vi "Online_Program.vi"() -> ()   [LabVIEW 2014]
uses:
  <vilib>/Utility/file.llb/Read From Spreadsheet File (DBL).vi
  <vilib>/Analysis/Matrix/Numeric/Conversions/Array To Matrix - RA2.vi
  <vilib>/Analysis/Matrix/Numeric/Conversions/Array To Matrix - RA.vi
  <vilib>/Utility/file.llb/Write To Spreadsheet File (DBL).vi
  <vilib>/Utility/file.llb/Write To Spreadsheet File (I64).vi
  <vilib>/Analysis/Matrix/NI_Matrix.lvlib
  <vilib>/Instr/_visa.llb/VISA Configure Serial Port (Instr).vi
  NeuroSky_Dll_Call/Debug/NeuroSky_Dll_Call.dll
panel:
  out "에러 출력":errorcluster
  out "메시지 2":string
  out "큐사인":bool
  out "icon_온도":bool
  out "icon_용변":bool
  out "icon_자판":bool
  out "icon_응급":bool=TRUE
  out "icon_기계":bool
  out "icon_침대":bool
  out "메시지":string
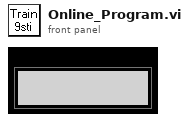
[diagram p1: front panel]
types:
  T1 = typedef "NI_Matrix.lvlib/RealMatrix.ctl" = dbl[][]
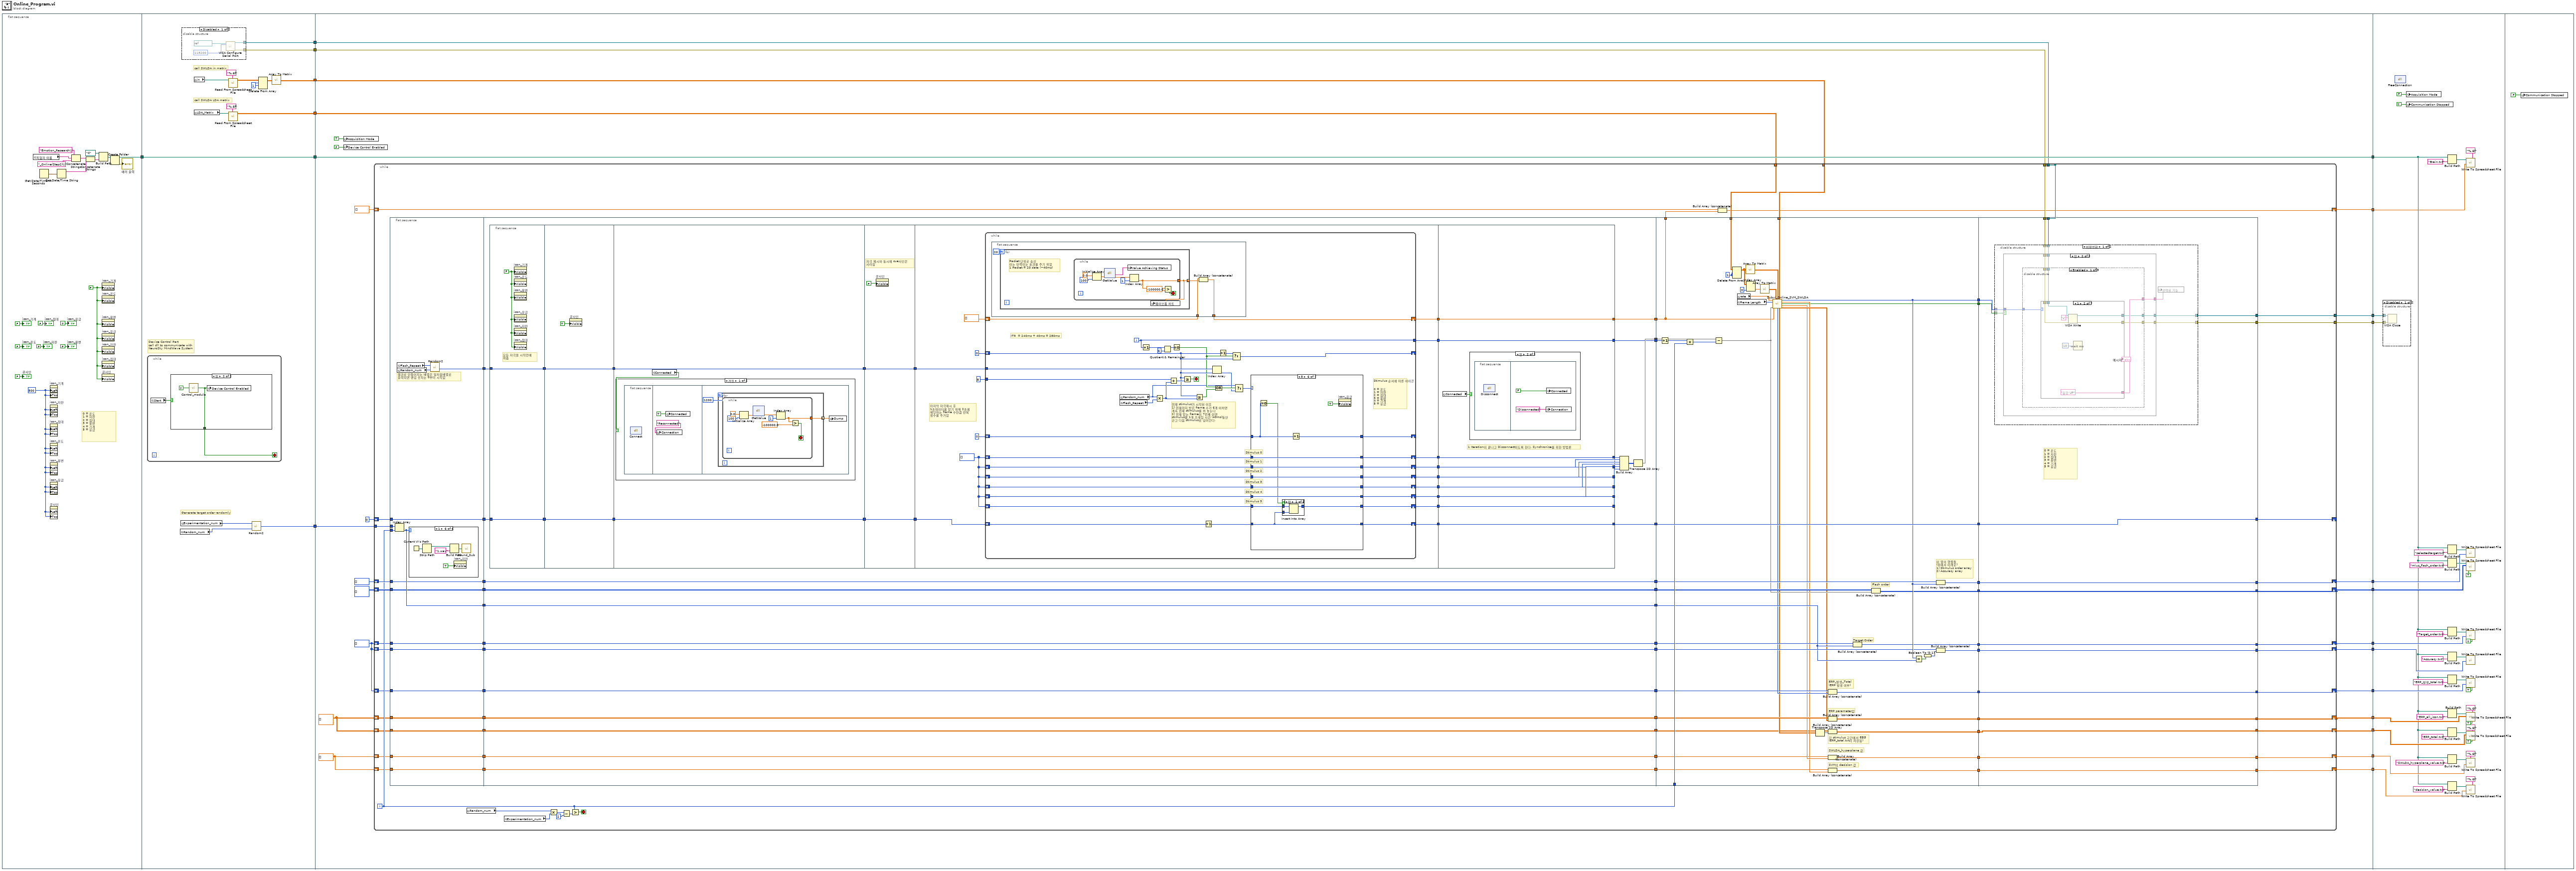
[diagram p0: block diagram]
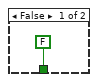
[diagram p3: hidden frame]
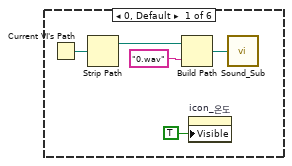
[diagram p4: hidden frame]
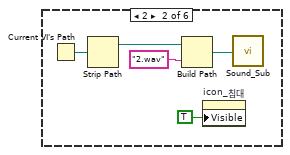
[diagram p5: hidden frame]
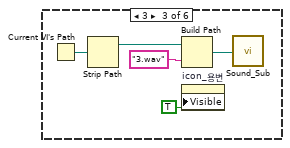
[diagram p6: hidden frame]
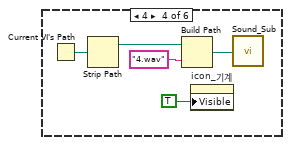
[diagram p7: hidden frame]
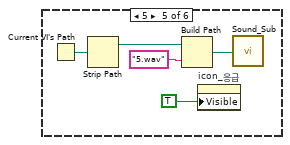
[diagram p8: hidden frame]
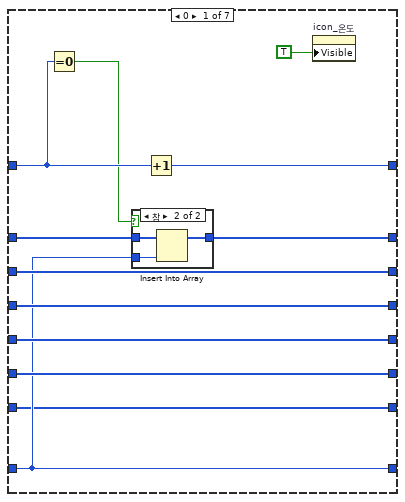
[diagram p10: hidden frame]
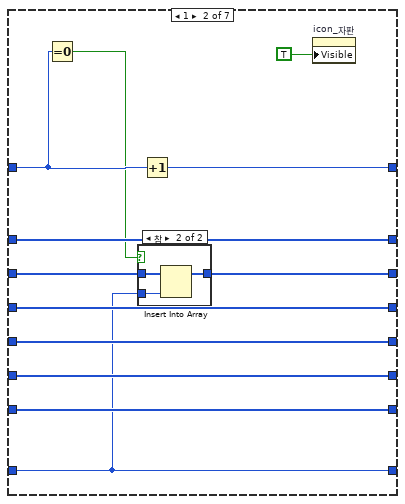
[diagram p12: hidden frame]
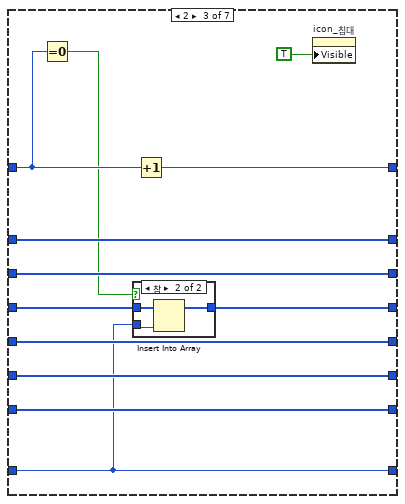
[diagram p14: hidden frame]
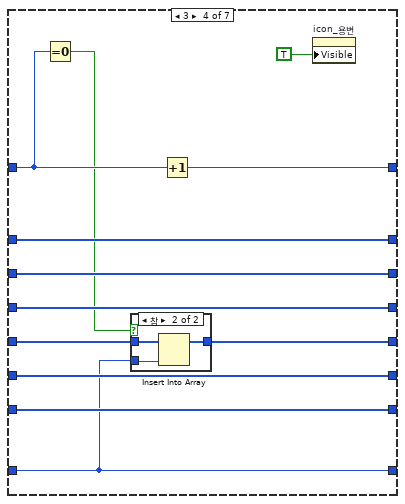
[diagram p16: hidden frame]
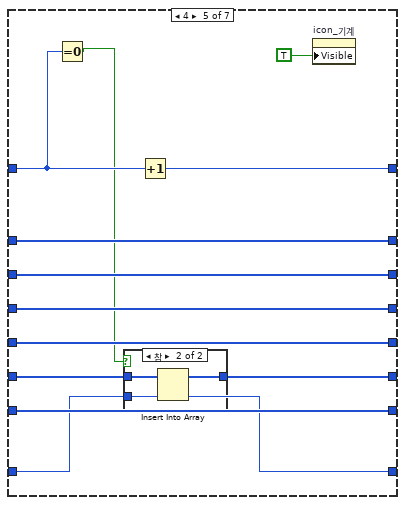
[diagram p18: hidden frame]
diagram:
  n1 = flat-sequence {
    tunnel: [w40] -> w20
    tunnel: w20 -> [w55]
    tunnel: [w55] -> w19
    tunnel: [w53] -> w18
    tunnel: [w49] -> w13
    tunnel: [w43] -> w7
    tunnel: [w42] -> w4
    tunnel: [w41] -> w3
    tunnel: w19 -> [w81]
    tunnel: [w81] -> w17
    tunnel: [w91] -> w16
    tunnel: [w89] -> w15
    tunnel: [w87] -> w14
    tunnel: w18 -> [w70]
    tunnel: w13 -> [w86]
    tunnel: [w85] -> w12
    tunnel: [w82] -> w11
    tunnel: [w78] -> w10
    tunnel: [w76] -> w9
    tunnel: [w75] -> w8
    tunnel: w7 -> [w69]
    tunnel: [w73] -> w6
    tunnel: [w71] -> w5
    tunnel: w4 -> [w68]
    tunnel: w3 -> [w67]
    tunnel: [w66] -> w2
    tunnel: [w65] -> w1
    tunnel: w17 -> [w663]
    tunnel: w16 -> [w658]
    tunnel: w15 -> [w697]
    tunnel: w14 -> [w693]
    tunnel: w12 -> [w690]
    tunnel: w11 -> [w686]
    tunnel: w10 -> [w680]
    tunnel: w9 -> [w675]
    tunnel: w8 -> [w672]
    tunnel: w6 -> [w669]
    tunnel: w5 -> [w664]
    tunnel: w2 -> [w660]
    tunnel: w1 -> [w659]
    frame #0 {
      w22 = FALSE ("Visible")
      w23 = 500 ("Position:Left")
      # "0 = 온도\n1 = 자판\n2 = 침대\n3 = 용변 \n4 = 기계 \n5 = 응급"
      n2 = global read "Control_Panel_정리.vi" "피험자 이름"() -> (w31:string)
      n3 = Get Date/Time In Seconds() -> (seconds since 1Jan1904=w37:timestamp)
      n4 = property on="icon_기계" class="Bool (엄격한)"("Left"=w23, "Top"=w23) -> ()  [unwired: 2 in, 2 out]
      n5 = property on="icon_자판" class="Bool (엄격한)"("Left"=w23, "Top"=w23) -> ()  [unwired: 2 in, 2 out]
      n6 = property on="icon_침대" class="Bool (엄격한)"("Left"=w23, "Top"=w23) -> ()  [unwired: 2 in, 2 out]
      n7 = property on="icon_온도" class="Bool (엄격한)"("Left"=w23, "Top"=w23) -> ()  [unwired: 2 in, 2 out]
      n8 = property on="icon_용변" class="Bool (엄격한)"("Left"=w23, "Top"=w23) -> ()  [unwired: 2 in, 2 out]
      n9 = property on="icon_응급" class="Bool (엄격한)"("Left"=w23, "Top"=w23) -> ()  [unwired: 2 in, 2 out]
      n10 = property on="큐사인" class="Bool (엄격한)"("Left"=w23, "Top"=w23) -> ()  [unwired: 2 in, 2 out]
      n11 = Get Date/Time String(seconds (now)=w37) -> (date string=w38:string)  [unwired: 2 in, 1 out]
      n12 = Concatenate Strings("Emotion_Research\\" ("string"), w31, "_Online(Step2)\\" ("문자열")) -> (w33:string)
      n13 = Concatenate Strings(w33, w38) -> (w35:string)
      n14 = Build Path(base path=path "C:/" ("path"), name or relative path=w35) -> (appended path=w36:path)
      n15 = property on="icon_기계" class="Bool (엄격한)"("Visible"=w22) -> ()  [unwired: 2 in, 2 out]
      n16 = property on="icon_온도" class="Bool (엄격한)"("Visible"=w22) -> ()  [unwired: 2 in, 2 out]
      n17 = property on="icon_용변" class="Bool (엄격한)"("Visible"=w22) -> ()  [unwired: 2 in, 2 out]
      n18 = property on="icon_응급" class="Bool (엄격한)"("Visible"=w22) -> ()  [unwired: 2 in, 2 out]
      n19 = property on="icon_자판" class="Bool (엄격한)"("Visible"=w22) -> ()  [unwired: 2 in, 2 out]
      n20 = property on="icon_침대" class="Bool (엄격한)"("Visible"=w22) -> ()  [unwired: 2 in, 2 out]
      n21 = property on="큐사인" class="Bool (엄격한)"("Visible"=w22) -> ()  [unwired: 2 in, 2 out]
      n22 = Create Folder(path (use dialog)=w36) -> (created path=w40:path, error out=→"에러 출력":errorcluster)  [unwired: 2 in, 1 out]
      "icon_온도" <- FALSE ("icon_전원 6")
      "icon_용변" <- FALSE ("icon_전체종료")
      "icon_자판" <- FALSE ("icon_음량업 2")
      "icon_응급" <- TRUE ("icon_채널다운")
      "icon_기계" <- FALSE ("icon_음량다")
      "icon_침대" <- FALSE ("icon_채널업")
      "큐사인" <- FALSE ("icon_전원 7")
    }
    frame #1 {
      w46 = 1 ("인덱스 (행)")
      # "call SWLDA in matrix"
      # "call SWLDA LDA matrix"
      # "Generate target order randomly"
      # "Device Control Part\ncall dll to communicate with\nNeuroSky MindWave System"
      n23 = while {
        stop <- w61 stop-if-true
        n24 = global read "Control_Panel_정리.vi" "Start"() -> (w60:bool)
        n25 = case shown="참" w60 {
          tunnel: [FALSE ("Connected") w63] -> w61
          frame False {
          }
          frame True {
            n26 = call "Control_module.vi"("Turn on"=TRUE ("Device Control Enabled")) -> ("Connected"=w63:bool)
            n27 = global write "Control_Panel_정리.vi" "Device Control Enabled"(w63) -> ()
          }
        }
      }
      n28 = global read "Control_Panel_정리.vi" "Random_num"() -> (w50:i32)
      n29 = global read "Control_Panel_정리.vi" "Experimentation_num"() -> (w51:i32)
      n30 = disable-structure shown="Disabled" {
        disable-tunnel: [w57 _] -> w42
        disable-tunnel: [w56 _] -> w41
        frame Disabled {
          n31 = call-poly "VISA Configure Serial Port"("VISA resource name"=refnum<visa-resource-name> "COM3", "baud rate (9600)"=u32 115200) -> ("VISA resource name out"=w57:refnum<visa-resource-name>, "error out"=w56:errorcluster)  [unwired: 12 in]
        }
        frame Enabled {
        }
      }
      n32 = global read "Control_Panel_정리.vi" "in"() -> (w44:path)
      n33 = global read "Control_Panel_정리.vi" "LDA_Matrix"() -> (w52:path)
      n34 = call-poly <vilib>:"Read From Spreadsheet File.vi"("format (%.3f)"="%.6f", "file path (dialog if empty)"=w44) -> ("all rows"=w45:dbl[][])  [unwired: 5 in, 4 out]
      n35 = call-poly <vilib>:"Read From Spreadsheet File.vi"("format (%.3f)"="%.6f", "file path (dialog if empty)"=w52) -> ("all rows"=w53:dbl[][])  [unwired: 5 in, 4 out]
      n36 = call "Random2.vi"("Random_num"=w50, "전체횟수"=w51) -> ("배열"=w49:i32[])
      n37 = Delete From Array(array=w45, length=w46, index (row)=w46) -> (array with subset deleted=w47:dbl[][])  [unwired: 1 in, 1 out]
      n38 = call-poly <vilib>:"Array To Matrix.vi"("Real 2D Array"=w47) -> ("Real Matrix"=w43:T1)
    }
    frame #2 {
      w74 = dbl[] []
      w72 = dbl[][] []
      w77 = i16[] []
      n39 = global write "Control_Panel_정리.vi" "Acquisition Mode"(TRUE ("Device Control Enabled")) -> ()
      n40 = global write "Control_Panel_정리.vi" "Device Control Enabled"(FALSE ("Device Control Enabled")) -> ()
      n41 = while {
        shift-right: [w92] -> w91
        shift-left: dbl[] [] -> [w100]
        shift-right: [w159] -> _
        shift-left: 0 ("y") -> [w165]
        shift-right: [w134] -> w89
        shift-left: i32[][] [] -> [w137]
        shift-right: [w143] -> w87
        shift-left: i32[] [] -> [w147]
        tunnel: w86 -> [w156]
        shift-right: [w138] -> w85
        shift-left: w77 -> [w142]
        shift-right: [w127] -> w82
        shift-left: w77 -> [w129]
        shift-right: [w125] -> w78
        shift-left: w77 -> [w124]
        shift-right: [w120] -> w76
        shift-left: w72 -> [w119]
        shift-right: [w115] -> w75
        shift-left: w74 -> [w114]
        shift-right: [w110] -> w73
        shift-left: w74 -> [w109]
        shift-right: [w105] -> w71
        shift-left: w72 -> [w104]
        tunnel: w70 -> [w101]
        tunnel: w69 -> [w98]
        tunnel: [w95] -> _
        tunnel: w68 -> [w95]
        tunnel: w67 -> [w96]
        tunnel: [w94] -> w66
        tunnel: [w93] -> w65
        i -> [w132]
        stop <- w148 stop-if-true
        n42 = flat-sequence {
          tunnel: [w182] -> w166
          tunnel: w165 -> [w181]
          tunnel: [w181] -> w164
          tunnel: w156 -> [w180]
          tunnel: w132 -> [w179]
          tunnel: [w176] -> w155
          tunnel: w147 -> [w175]
          tunnel: [w175] -> w146
          tunnel: w142 -> [w174]
          tunnel: [w174] -> w140
          tunnel: w137 -> [w173]
          tunnel: [w173] -> w135
          tunnel: [w172] -> w130
          tunnel: w129 -> [w172]
          tunnel: w124 -> [w171]
          tunnel: [w171] -> w122
          tunnel: w119 -> [w170]
          tunnel: [w170] -> w117
          tunnel: w114 -> [w169]
          tunnel: [w169] -> w112
          tunnel: w109 -> [w168]
          tunnel: [w168] -> w107
          tunnel: w104 -> [w167]
          tunnel: [w167] -> w103
          tunnel: w166 -> [w252]
          tunnel: w164 -> [w249]
          tunnel: [w250] -> w163
          tunnel: [w239] -> w162
          tunnel: [w248] -> w161
          tunnel: [w247] -> w160
          tunnel: w155 -> [w246]
          tunnel: [w246] -> w154
          tunnel: w146 -> [w245]
          tunnel: [w245] -> w145
          tunnel: [w244] -> w141
          tunnel: w140 -> [w244]
          tunnel: [w243] -> w136
          tunnel: w135 -> [w243]
          tunnel: [w242] -> w131
          tunnel: w130 -> [w242]
          tunnel: [w241] -> w123
          tunnel: w122 -> [w241]
          tunnel: [w240] -> w118
          tunnel: w117 -> [w240]
          tunnel: [w238] -> w113
          tunnel: w112 -> [w238]
          tunnel: [w237] -> w108
          tunnel: w107 -> [w237]
          tunnel: w103 -> [w236]
          tunnel: [w236] -> w102
          tunnel: w163 -> [w491]
          tunnel: w162 -> [w465]
          tunnel: w161 -> [w505]
          tunnel: w160 -> [w506]
          tunnel: w132 -> [w504]
          tunnel: [w505] -> w158
          tunnel: [w499] -> w157
          tunnel: w154 -> [w490]
          tunnel: w145 -> [w500]
          tunnel: [w498] -> w144
          tunnel: w141 -> [w496]
          tunnel: [w495] -> w139
          tunnel: w136 -> [w494]
          tunnel: [w492] -> w133
          tunnel: w131 -> [w489]
          tunnel: [w488] -> w128
          tunnel: [w486] -> w126
          tunnel: w123 -> [w485]
          tunnel: [w483] -> w121
          tunnel: w118 -> [w482]
          tunnel: [w480] -> w116
          tunnel: w113 -> [w479]
          tunnel: [w477] -> w111
          tunnel: w108 -> [w476]
          tunnel: [w473] -> w106
          tunnel: w102 -> [w472]
          tunnel: w101 -> [w471]
          tunnel: [w465] -> w99
          tunnel: w98 -> [w467]
          tunnel: [w466] -> w97
          tunnel: [w527] -> w159
          tunnel: [w526] -> w143
          tunnel: [w523] -> w138
          tunnel: [w525] -> w134
          tunnel: [w524] -> w127
          tunnel: [w522] -> w125
          tunnel: [w521] -> w120
          tunnel: [w520] -> w115
          tunnel: [w519] -> w110
          tunnel: [w518] -> w105
          tunnel: w106 -> [w518]
          tunnel: w111 -> [w519]
          tunnel: w116 -> [w520]
          tunnel: w121 -> [w521]
          tunnel: w126 -> [w522]
          tunnel: w128 -> [w524]
          tunnel: w133 -> [w525]
          tunnel: w139 -> [w523]
          tunnel: w144 -> [w526]
          tunnel: w157 -> [w517]
          tunnel: w158 -> [w527]
          tunnel: w97 -> [w516]
          tunnel: w96 -> [w515]
          tunnel: w95 -> [w514]
          tunnel: [w513] -> w94
          tunnel: [w512] -> w93
          frame #0 {
            # "결과로 만들어지는 배열은 일차원배열로\n출력되면 랜덤 숫자는 0부터 시작함"
            n43 = Index Array(array=w180, index=w179) -> (element=w176:i32)
            n44 = global read "Control_Panel_정리.vi" "Flash_Repeat"() -> (w178:i32)
            n45 = global read "Control_Panel_정리.vi" "Random_num"() -> (w177:i32)
            n46 = case shown="1" w176 {
              frame 0, Default {
                n47 = Current VI's Path() -> (path=w185:path)
                n48 = Strip Path(path=w185) -> (stripped path=w186:path)  [unwired: 1 out]
                n49 = Build Path(base path=w186, name or relative path="0.wav" ("이름 또는 상대 경로")) -> (appended path=w184:path)
                n50 = property on="icon_온도" class="Bool (엄격한)"("Visible"=TRUE) -> ()  [unwired: 2 in, 2 out]
                n51 = call "Sound_Sub.vi"("path"=w184) -> ()
              }
              frame 2 {
                n52 = Current VI's Path() -> (path=w189:path)
                n53 = Strip Path(path=w189) -> (stripped path=w190:path)  [unwired: 1 out]
                n54 = Build Path(base path=w190, name or relative path="2.wav" ("이름 또는 상대 경로")) -> (appended path=w192:path)
                n55 = property on="icon_침대" class="Bool (엄격한)"("Visible"=TRUE) -> ()  [unwired: 2 in, 2 out]
                n56 = call "Sound_Sub.vi"("path"=w192) -> ()
              }
              frame 3 {
                n57 = Current VI's Path() -> (path=w194:path)
                n58 = Strip Path(path=w194) -> (stripped path=w195:path)  [unwired: 1 out]
                n59 = Build Path(base path=w195, name or relative path="3.wav" ("이름 또는 상대 경로")) -> (appended path=w197:path)
                n60 = property on="icon_용변" class="Bool (엄격한)"("Visible"=TRUE) -> ()  [unwired: 2 in, 2 out]
                n61 = call "Sound_Sub.vi"("path"=w197) -> ()
              }
              frame 4 {
                n62 = Current VI's Path() -> (path=w199:path)
                n63 = Strip Path(path=w199) -> (stripped path=w200:path)  [unwired: 1 out]
                n64 = Build Path(base path=w200, name or relative path="4.wav" ("이름 또는 상대 경로")) -> (appended path=w202:path)
                n65 = property on="icon_기계" class="Bool (엄격한)"("Visible"=TRUE) -> ()  [unwired: 2 in, 2 out]
                n66 = call "Sound_Sub.vi"("path"=w202) -> ()
              }
              frame 5 {
                n67 = Current VI's Path() -> (path=w204:path)
                n68 = Strip Path(path=w204) -> (stripped path=w205:path)  [unwired: 1 out]
                n69 = Build Path(base path=w205, name or relative path="5.wav" ("이름 또는 상대 경로")) -> (appended path=w207:path)
                n70 = property on="icon_응급" class="Bool (엄격한)"("Visible"=TRUE) -> ()  [unwired: 2 in, 2 out]
                n71 = call "Sound_Sub.vi"("path"=w207) -> ()
              }
              frame 1 {
                n72 = Current VI's Path() -> (path=w210:path)
                n73 = Strip Path(path=w210) -> (stripped path=w211:path)  [unwired: 1 out]
                n74 = Build Path(base path=w211, name or relative path="1.wav" ("이름 또는 상대 경로")) -> (appended path=w209:path)
                n75 = property on="icon_자판" class="Bool (엄격한)"("Visible"=TRUE) -> ()  [unwired: 2 in, 2 out]
                n76 = call "Sound_Sub.vi"("path"=w209) -> ()
              }
            }
            n77 = call "Random2.vi"("Random_num"=w177, "전체횟수"=w178) -> ("배열"=w182:i32[])
          }
          frame #1 {
            n78 = flat-sequence {
              tunnel: w249 -> [w254]
              tunnel: w252 -> [w255]
              tunnel: [w255] -> w235
              tunnel: [w254] -> w234
              tunnel: [w258] -> w227
              tunnel: [w257] -> w226
              tunnel: w235 -> [w258]
              tunnel: w234 -> [w257]
              tunnel: w227 -> [w261]
              tunnel: [w261] -> w216
              tunnel: w226 -> [w260]
              tunnel: [w260] -> w214
              tunnel: w216 -> [w277]
              tunnel: [w277] -> w215
              tunnel: w214 -> [w276]
              tunnel: [w276] -> w213
              tunnel: w215 -> [w293]
              tunnel: w213 -> [w283]
              tunnel: [w291] -> w225
              tunnel: [w290] -> w224
              tunnel: [w289] -> w223
              tunnel: [w288] -> w222
              tunnel: [w287] -> w221
              tunnel: [w282] -> w220
              tunnel: [w281] -> w219
              tunnel: [w280] -> w218
              tunnel: [w278] -> w217
              tunnel: [w454] -> w239
              tunnel: [w455] -> w230
              tunnel: [w456] -> w247
              tunnel: [w457] -> w248
              tunnel: [w458] -> w233
              tunnel: [w459] -> w232
              tunnel: [w460] -> w231
              tunnel: [w461] -> w229
              tunnel: [w462] -> w228
              tunnel: w225 -> [w462]
              tunnel: w224 -> [w461]
              tunnel: w223 -> [w460]
              tunnel: w222 -> [w459]
              tunnel: w221 -> [w458]
              tunnel: w220 -> [w457]
              tunnel: w219 -> [w456]
              tunnel: w218 -> [w455]
              tunnel: w217 -> [w454]
              frame #0 {
                w253 = FALSE ("Visible")
                # "모든 자극을 시작전에\n꺼줌"
                n79 = property on="icon_기계" class="Bool (엄격한)"("Visible"=w253) -> ()  [unwired: 2 in, 2 out]
                n80 = property on="icon_온도" class="Bool (엄격한)"("Visible"=w253) -> ()  [unwired: 2 in, 2 out]
                n81 = property on="icon_용변" class="Bool (엄격한)"("Visible"=w253) -> ()  [unwired: 2 in, 2 out]
                n82 = property on="icon_응급" class="Bool (엄격한)"("Visible"=w253) -> ()  [unwired: 2 in, 2 out]
                n83 = property on="icon_자판" class="Bool (엄격한)"("Visible"=w253) -> ()  [unwired: 2 in, 2 out]
                n84 = property on="icon_침대" class="Bool (엄격한)"("Visible"=w253) -> ()  [unwired: 2 in, 2 out]
              }
              frame #1 {
                n85 = property on="큐사인" class="Bool (엄격한)"("Visible"=TRUE) -> ()  [unwired: 2 in, 2 out]
              }
              frame #2 {
                n86 = global read "Control_Panel_정리.vi" "Connected"() -> (w259:bool)
                n87 = case shown="거짓" w259 {
                  frame False {
                    n88 = flat-sequence {
                      frame #0 {
                        n89 = dll-call lib="C:/Users/Server/Desktop/NeuroSky/NeuroSky_Dll_Call/Debug/NeuroSky_Dll_Call.dll" fn="Connect"() -> ()  [unwired: 4 in, 2 out]
                      }
                      frame #1 {
                        n90 = global write "Control_Panel_정리.vi" "Connection"("Reconnected") -> ()
                        n91 = global write "Control_Panel_정리.vi" "Connected"(TRUE ("Connected")) -> ()
                      }
                      frame #2 {
                        n92 = for {
                          N: 1200 -> [_]
                          tunnel: [w266] -> w264 mode=indexing
                          n93 = while {
                            tunnel: [w268] -> w266
                            stop <- w267 stop-if-true
                            n94 = Initialize Array(0.0 ("element"), 100 ("dimension size")) -> (w273:dbl[])
                            n95 = dll-call lib="C:/Users/Server/Desktop/NeuroSky/NeuroSky_Dll_Call/Debug/NeuroSky_Dll_Call.dll" fn="GetValue"("result"=w273) -> ("result"=w274:dbl[])  [unwired: 4 in, 2 out]
                            n96 = Index Array(array=w274, index=1) -> (element=w268:dbl)
                            n97 = Greater?(x=w268, y=-100000.0) -> (0:w267:bool)
                          }
                        }
                        n98 = global write "Control_Panel_정리.vi" "Dump"(w264) -> ()
                      }
                    }
                  }
                  frame True {
                  }
                }
              }
              frame #3 {
                # "자극 제시와 동시에 cue사인은\n사라짐"
                n99 = property on="큐사인" class="Bool (엄격한)"("Visible"=FALSE) -> ()  [unwired: 2 in, 2 out]
              }
              frame #4 {
                w285 = i32[] []
                # "마지막 자극제시 후\n1초데이터를 받기 위해 2초에\n해당하는 frame 수만큼 반복\n횟수를 추가함"
                n100 = while {
                  tunnel: w293 -> [w329]
                  shift-right: [w297] -> w278
                  shift-left: dbl[] [] -> [w298]
                  tunnel: 8 -> [w294]
                  shift-right: [w326] -> w291
                  shift-left: w285 -> [w325]
                  shift-right: [w323] -> w290
                  shift-left: w285 -> [w324]
                  shift-right: [w321] -> w280
                  shift-left: w285 -> [w322]
                  shift-right: [w319] -> w289
                  shift-left: w285 -> [w320]
                  shift-right: [w317] -> w288
                  shift-left: w285 -> [w318]
                  shift-right: [w316] -> w287
                  shift-left: w285 -> [w303]
                  shift-right: [w314] -> w282
                  shift-left: w283 -> [w315]
                  shift-right: [w310] -> _
                  shift-left: 0 -> [w309]
                  shift-right: [w304] -> _
                  shift-left: 0 ("y") -> [w305]
                  tunnel: [w299] -> w281
                  i -> [w299]
                  stop <- w330 stop-if-true
                  # "ITR  = 240ms + 40ms = 280ms"
                  # "현재 stimulus가 시작된 이후\n1) 현재까지 받은 frame 수가 6개 이하면\n계속 현재 stimulus를 켜 놓는다\n2) 현재 받는 frame이 7번째 이면\nstimulus를 1개 프레임 시간 (40ms)동안\n끈고 다음 stimulus로 넘어간다."
                  # "Stimulus 순서에 따른 아이콘\n\n\n0 = 온도\n1 = 자판\n2 = 침대\n3 = 용변 \n4 = 기계 \n5 = 응급"
                  # "Stimulus 5"
                  # "Stimulus 4"
                  # "Stimulus 3"
                  # "Stimulus 2"
                  # "Stimulus 1"
                  # "Stimulus 0"
                  n101 = flat-sequence {
                    tunnel: [w335] -> w297
                    tunnel: w298 -> [w334]
                    frame #0 {
                      n102 = for {
                        N: 20 -> [_]
                        tunnel: [w336] -> w333 mode=indexing
                        # "Packet 단위로 송신\n이는 반짝이는 효과를 주기 위함\n1 Packet = 20 data (~40ms)"
                        n103 = while {
                          tunnel: [w338] -> w336
                          stop <- w337 stop-if-true
                          n104 = Initialize Array(0.0 ("element"), 100 ("dimension size")) -> (w344:dbl[])
                          n105 = dll-call lib="C:/Users/Server/Desktop/NeuroSky/NeuroSky_Dll_Call/Debug/NeuroSky_Dll_Call.dll" fn="GetValue"("result"=w344) -> ("errCode"=w340:string, "result"=w345:dbl[])  [unwired: 3 in, 2 out]
                          n106 = global write "Control_Panel_정리.vi" "Value Achieving Status"(w340) -> ()
                          n107 = Index Array(array=w345, index=1) -> (element=w338:dbl)
                          n108 = Greater?(x=w338, y=-100000.0) -> (0:w337:bool)
                        }
                        n109 = global write "Control_Panel_정리.vi" "웨이브폼 차트"(w336) -> ()
                      }
                      n110 = Build Array (concatenate)(w334, w333) -> (w335:dbl[])
                    }
                  }
                  n111 = global read "Control_Panel_정리.vi" "Random_num"() -> (w296:i32)
                  n112 = global read "Control_Panel_정리.vi" "Flash_Repeat"() -> (w295:i32)
                  n113 = Increment(x=w299) -> (x+1=w302:i32)
                  n114 = Multiply(x=w296, y=w295) -> (x*y=w300:i32)
                  n115 = Quotient & Remainder(x=w302, y=6) -> (x-y*floor(x/y)=w312:i32)  [unwired: 1 out]
                  n116 = Add(x=w294, y=w300) -> (x+y=w331:i32)
                  n117 = Equal To 0?(x=w312) -> (x = 0?=w308:bool)
                  n118 = Greater Or Equal?(x=w309, y=w331) -> (x >= y?=w330:bool)
                  n119 = Greater Or Equal?(x=w309, y=w300) -> (x >= y?=w307:bool)
                  n120 = Increment(x=w315) -> (x+1=w327:i32)
                  n121 = Index Array(array=w329, index=w309) -> (element=w301:i32)
                  n122 = Or(x=w308, y=w307) -> (x .or. y?=w306:bool)
                  n123 = Increment(x=w309) -> (x+1=w311:i32)
                  n124 = Select(t=w311, s=w308, f=w309) -> (s? t:f=w310:i32)
                  n125 = Select(t=w296, s=w306, f=w301) -> (s? t:f=w328:i32)
                  n126 = case shown="5" w328 {
                    tunnel: w327 -> [w351 w367 w382 w398 w414 w431 w446]
                    tunnel: [w356 w364 w389 w405 w421 w437 w452] -> w326
                    tunnel: w325 -> [w357 w364 w389 w405 w421 w437 w452]
                    tunnel: w324 -> [w355 w373 w386 w402 w418 w435 w451]
                    tunnel: [w355 w372 w386 w402 w418 w435 w451] -> w323
                    tunnel: w322 -> [w354 w371 w388 w401 w417 w434 w450]
                    tunnel: [w354 w371 w387 w401 w417 w434 w450] -> w321
                    tunnel: w320 -> [w353 w370 w385 w404 w416 w433 w449]
                    tunnel: [w353 w370 w385 w403 w416 w433 w449] -> w319
                    tunnel: w318 -> [w352 w369 w384 w400 w420 w432 w448]
                    tunnel: [w352 w369 w384 w400 w419 w432 w448] -> w317
                    tunnel: w303 -> [w348 w368 w383 w399 w415 w436 w447]
                    tunnel: [w348 w368 w383 w399 w415 w428 w447] -> w316
                    tunnel: [w351 w367 w382 w398 w414 w431 w446] -> w314
                    tunnel: w305 -> [w350 w366 w381 w396 w413 w429 _]
                    tunnel: [w349 w365 w380 w397 w412 w430 0] -> w304
                    frame 0 {
                      n127 = Equal To 0?(x=w350) -> (x = 0?=w346:bool)
                      n128 = case shown="참" w346 {
                        tunnel: w357 -> [w358 w361]
                        tunnel: [w358 w360] -> w356
                        tunnel: w351 -> [_ w359]
                        frame False {
                        }
                        frame True {
                          n129 = Insert Into Array(array=w361, new element=w359) -> (w360:i32[])  [unwired: 1 in]
                        }
                      }
                      n130 = Increment(x=w350) -> (x+1=w349:i32)
                      n131 = property on="icon_온도" class="Bool (엄격한)"("Visible"=TRUE) -> ()  [unwired: 2 in, 2 out]
                    }
                    frame 1 {
                      n132 = Equal To 0?(x=w366) -> (x = 0?=w362:bool)
                      n133 = case shown="참" w362 {
                        tunnel: w373 -> [w374 w377]
                        tunnel: [w374 w376] -> w372
                        tunnel: w367 -> [_ w375]
                        frame False {
                        }
                        frame True {
                          n134 = Insert Into Array(array=w377, new element=w375) -> (w376:i32[])  [unwired: 1 in]
                        }
                      }
                      n135 = Increment(x=w366) -> (x+1=w365:i32)
                      n136 = property on="icon_자판" class="Bool (엄격한)"("Visible"=TRUE) -> ()  [unwired: 2 in, 2 out]
                    }
                    frame 2 {
                      n137 = Equal To 0?(x=w381) -> (x = 0?=w378:bool)
                      n138 = case shown="참" w378 {
                        tunnel: w388 -> [w390 w393]
                        tunnel: [w390 w392] -> w387
                        tunnel: w382 -> [_ w391]
                        frame False {
                        }
                        frame True {
                          n139 = Insert Into Array(array=w393, new element=w391) -> (w392:i32[])  [unwired: 1 in]
                        }
                      }
                      n140 = Increment(x=w381) -> (x+1=w380:i32)
                      n141 = property on="icon_침대" class="Bool (엄격한)"("Visible"=TRUE) -> ()  [unwired: 2 in, 2 out]
                    }
                    frame 3 {
                      n142 = Equal To 0?(x=w396) -> (x = 0?=w394:bool)
                      n143 = case shown="참" w394 {
                        tunnel: w404 -> [w406 w409]
                        tunnel: [w406 w408] -> w403
                        tunnel: w398 -> [_ w407]
                        frame False {
                        }
                        frame True {
                          n144 = Insert Into Array(array=w409, new element=w407) -> (w408:i32[])  [unwired: 1 in]
                        }
                      }
                      n145 = Increment(x=w396) -> (x+1=w397:i32)
                      n146 = property on="icon_용변" class="Bool (엄격한)"("Visible"=TRUE) -> ()  [unwired: 2 in, 2 out]
                    }
                    frame 4 {
                      n147 = Equal To 0?(x=w413) -> (x = 0?=w410:bool)
                      n148 = case shown="참" w410 {
                        tunnel: w420 -> [w422 w425]
                        tunnel: [w422 w424] -> w419
                        tunnel: w414 -> [_ w423]
                        frame False {
                        }
                        frame True {
                          n149 = Insert Into Array(array=w425, new element=w423) -> (w424:i32[])  [unwired: 1 in]
                        }
                      }
                      n150 = Increment(x=w413) -> (x+1=w412:i32)
                      n151 = property on="icon_기계" class="Bool (엄격한)"("Visible"=TRUE) -> ()  [unwired: 2 in, 2 out]
                    }
                    frame 5 {
                      n152 = Equal To 0?(x=w429) -> (x = 0?=w426:bool)
                      n153 = case shown="참" w426 {
                        tunnel: w436 -> [w438 w441]
                        tunnel: [w438 w440] -> w428
                        tunnel: w431 -> [_ w439]
                        frame False {
                        }
                        frame True {
                          n154 = Insert Into Array(array=w441, new element=w439) -> (w440:i32[])  [unwired: 1 in]
                        }
                      }
                      n155 = Increment(x=w429) -> (x+1=w430:i32)
                      n156 = property on="icon_응급" class="Bool (엄격한)"("Visible"=TRUE) -> ()  [unwired: 2 in, 2 out]
                    }
                    frame 6, Default {
                      w443 = FALSE ("Visible")
                      w444 = FALSE ("Visible")
                      w442 = FALSE ("Visible")
                      n157 = property on="icon_기계" class="Bool (엄격한)"("Visible"=w442) -> ()  [unwired: 2 in, 2 out]
                      n158 = property on="icon_온도" class="Bool (엄격한)"("Visible"=w442) -> ()  [unwired: 2 in, 2 out]
                      n159 = property on="icon_응급" class="Bool (엄격한)"("Visible"=w444) -> ()  [unwired: 2 in, 2 out]
                      n160 = property on="icon_용변" class="Bool (엄격한)"("Visible"=w444) -> ()  [unwired: 2 in, 2 out]
                      n161 = property on="icon_자판" class="Bool (엄격한)"("Visible"=w443) -> ()  [unwired: 2 in, 2 out]
                      n162 = property on="icon_침대" class="Bool (엄격한)"("Visible"=w443) -> ()  [unwired: 2 in, 2 out]
                    }
                  }
                }
              }
              frame #5 {
                # "1 Iteration이 끝나고 Disconnect하도록 한다. Synchronize를 위한 방법론"
                n163 = global read "Control_Panel_정리.vi" "Connected"() -> (w453:bool)
                n164 = case shown="참" w453 {
                  frame False {
                  }
                  frame True {
                    n165 = flat-sequence {
                      frame #0 {
                        n166 = dll-call lib="C:/Users/Server/Desktop/NeuroSky/NeuroSky_Dll_Call/Debug/NeuroSky_Dll_Call.dll" fn="Disconnect"() -> ()  [unwired: 4 in, 2 out]
                      }
                      frame #1 {
                        n167 = global write "Control_Panel_정리.vi" "Connection"("Disconnected") -> ()
                        n168 = global write "Control_Panel_정리.vi" "Connected"(FALSE ("Connected")) -> ()
                      }
                    }
                  }
                }
              }
            }
            n169 = Build Array(w228, w229, w230, w231, w232, w233) -> (w251:i32[][])
            n170 = Transpose 2D Array(2D array=w251) -> (transposed array=w250:i32[][])
          }
          frame #2 {
            w509 = 1 ("인덱스 (행)")
            # "각 stimulus 구간에서 EEG\n(ERP_total.txt라 저장됨)"
            # "ERP parameter값"
            # "SVM의 decision 값"
            # "SWLDA_hyperplane 값"
            # "ERP_발생_Total\n(ERP 발생 여부)"
            # "Target Order"
            # "Flash order"
            # "이 열의 행렬들 \n(위에서 아래로)\n1) Stimulus order array\n2) Accuracy array"
            n171 = Increment(x=w506) -> (x+1=w510:i32)
            n172 = Multiply(x=w510, y=w504) -> (x*y=w511:i32)
            n173 = Subtract(x=w491, y=w511) -> (x-y=w493:i32[][])
            n174 = Delete From Array(array=w471, length=w509, index (row)=w509) -> (array with subset deleted=w469:dbl[][])  [unwired: 1 in, 1 out]
            n175 = global read "Control_Panel_정리.vi" "rate"() -> (w502:dbl)
            n176 = global read "Control_Panel_정리.vi" "Frame Length"() -> (w503:i32)
            n177 = call-poly <vilib>:"Array To Matrix.vi"("Real 2D Array"=w469) -> ("Real Matrix"=w468:T1)
            n178 = Index Array(array=w469, index (col)=0 ("인덱스")) -> (element=w470:dbl[])  [unwired: 1 in]
            n179 = call-poly <vilib>:"Array To Matrix.vi"("Real 1D Array"=w470) -> ("Real Matrix (Column Vector)"=w507:T1)
            n180 = call "Subvi_Online_SVM_SWLDA.vi"("rate"=w502, "Value"=w507, "Matrix"=w468, "in"=w467, "samples per channel"=w503, "Brain_data_source"=w465, "Target_Flash_Order"=w493) -> ("output-0~8"=w499:i32, "decision"=w478:dbl[], "ERP_발생여부"=w466:bool, "SWLDA"=w481:dbl[], "EPR_발생_total"=w487:i16[], "ERP_all"=w475:dbl[][], "ERP_Parameters"=w484:dbl[][])  [unwired: 2 in]
            n181 = Transpose 2D Array(2D array=w475) -> (transposed array=w474:dbl[][])
            n182 = Build Array (concatenate)(w485, w487) -> (w486:i16[])
            n183 = Build Array (concatenate)(w482, w484) -> (w483:dbl[][])
            n184 = Build Array (concatenate)(w472, w474) -> (w473:dbl[][])
            n185 = Build Array (concatenate)(w479, w481) -> (w480:dbl[])
            n186 = Build Array (concatenate)(w476, w478) -> (w477:dbl[])
            n187 = Build Array (concatenate)(w489, w490) -> (w488:i32[])
            n188 = Build Array (concatenate)(w494, w493) -> (w492:i32[][])
            n189 = Equal?(x=w499, y=w490) -> (x = y?=w501:bool)
            n190 = Boolean To (0,1)(Boolean=w501) -> (0, 1=w497:i16)
            n191 = Build Array (concatenate)(w500, w499) -> (w498:i32[])
            n192 = Build Array (concatenate)(w496, w497) -> (w495:i16[])
          }
          frame #3 {
            # "0 = 온도\n1 = 자판\n2 = 침대\n3 = 용변 \n4 = 기계 \n5 = 응급"
            n193 = disable-structure shown="비활성화" {
              disable-tunnel: w517 -> [w534 w619]
              disable-tunnel: w516 -> [w533 w618]
              disable-tunnel: w515 -> [w532 _]
              disable-tunnel: w514 -> [w531 _]
              disable-tunnel: [w530 _] -> w513
              disable-tunnel: [w529 _] -> w512
              frame Disabled {
                n194 = case shown="참" w533 {
                  tunnel: w534 -> [_ w543]
                  tunnel: ["No Decesion" ("메시지") w542] -> w528
                  tunnel: w532 -> [w535 w541]
                  tunnel: w531 -> [w536 w540]
                  tunnel: [w536 w539] -> w530
                  tunnel: [w535 w538] -> w529
                  frame False {
                  }
                  frame True {
                    n195 = disable-structure shown="Enabled" {
                      disable-tunnel: [w549 _ "" ("메시지")] -> w542
                      disable-tunnel: w543 -> [w548 w591 _]
                      disable-tunnel: w541 -> [w547 _ _]
                      disable-tunnel: w540 -> [w546 _ _]
                      disable-tunnel: [w545 _ _] -> w539
                      disable-tunnel: [w544 _ _] -> w538
                      frame Enabled {
                        n196 = case shown="1" w548 {
                          tunnel: ["전원" ("메시지") "음향 UP" ("메시지") "채널 UP" ("메시지") "전체종료" ("메시지") "음향 Down" ("메시지") "채널 Down" ("메시지") "No Decesion" ("메시지")] -> w549
                          tunnel: w547 -> [w553 w560 w566 w571 w577 w584 w588]
                          tunnel: w546 -> [w552 w559 w567 w572 w576 w583 w589]
                          tunnel: [w551 w558 w565 w572 w575 w582 w589] -> w545
                          tunnel: [w550 w557 w564 w571 w574 w581 w588] -> w544
                          frame 0 {
                            n197 = VISA Write(VISA resource name=w552, write buffer="0", error in (no error)=w553) -> (VISA resource name out=w551:refnum<visa-resource-name>, error out=w550:errorcluster)  [unwired: 1 out]
                            n198 = Wait (ms)(milliseconds to wait=u32 10) -> ()  [unwired: 1 out]
                          }
                          frame 1 {
                            n199 = VISA Write(VISA resource name=w559, write buffer="L", error in (no error)=w560) -> (VISA resource name out=w558:refnum<visa-resource-name>, error out=w557:errorcluster)  [unwired: 1 out]
                            n200 = Wait (ms)(milliseconds to wait=u32 10) -> ()  [unwired: 1 out]
                          }
                          frame 2 {
                            n201 = VISA Write(VISA resource name=w567, write buffer="J", error in (no error)=w566) -> (VISA resource name out=w565:refnum<visa-resource-name>, error out=w564:errorcluster)  [unwired: 1 out]
                            n202 = Wait (ms)(milliseconds to wait=u32 10) -> ()  [unwired: 1 out]
                          }
                          frame 3 {
                          }
                          frame 4 {
                            n203 = VISA Write(VISA resource name=w576, write buffer="M", error in (no error)=w577) -> (VISA resource name out=w575:refnum<visa-resource-name>, error out=w574:errorcluster)  [unwired: 1 out]
                            n204 = Wait (ms)(milliseconds to wait=u32 10) -> ()  [unwired: 1 out]
                          }
                          frame 5 {
                            n205 = VISA Write(VISA resource name=w583, write buffer="K", error in (no error)=w584) -> (VISA resource name out=w582:refnum<visa-resource-name>, error out=w581:errorcluster)  [unwired: 1 out]
                            n206 = Wait (ms)(milliseconds to wait=u32 10) -> ()  [unwired: 1 out]
                          }
                          frame 9, Default {
                          }
                        }
                      }
                      frame Disabled {
                        n207 = case shown="0, 기본" w591 {
                          frame 0, Default {
                            n208 = Current VI's Path() -> (path=w593:path)
                            n209 = Strip Path(path=w593) -> (stripped path=w594:path)  [unwired: 1 out]
                            n210 = Build Path(base path=w594, name or relative path="0.wav" ("이름 또는 상대 경로")) -> (appended path=w592:path)
                            n211 = call "Sound_Sub.vi"("path"=w592) -> ()
                          }
                          frame 2 {
                            n212 = Current VI's Path() -> (path=w596:path)
                            n213 = Strip Path(path=w596) -> (stripped path=w597:path)  [unwired: 1 out]
                            n214 = Build Path(base path=w597, name or relative path="2.wav" ("이름 또는 상대 경로")) -> (appended path=w599:path)
                            n215 = call "Sound_Sub.vi"("path"=w599) -> ()
                          }
                          frame 3 {
                            n216 = Current VI's Path() -> (path=w600:path)
                            n217 = Strip Path(path=w600) -> (stripped path=w601:path)  [unwired: 1 out]
                            n218 = Build Path(base path=w601, name or relative path="3.wav" ("이름 또는 상대 경로")) -> (appended path=w603:path)
                            n219 = call "Sound_Sub.vi"("path"=w603) -> ()
                          }
                          frame 4 {
                            n220 = Current VI's Path() -> (path=w604:path)
                            n221 = Strip Path(path=w604) -> (stripped path=w605:path)  [unwired: 1 out]
                            n222 = Build Path(base path=w605, name or relative path="4.wav" ("이름 또는 상대 경로")) -> (appended path=w607:path)
                            n223 = call "Sound_Sub.vi"("path"=w607) -> ()
                          }
                          frame 5 {
                            n224 = Current VI's Path() -> (path=w608:path)
                            n225 = Strip Path(path=w608) -> (stripped path=w609:path)  [unwired: 1 out]
                            n226 = Build Path(base path=w609, name or relative path="5.wav" ("이름 또는 상대 경로")) -> (appended path=w611:path)
                            n227 = call "Sound_Sub.vi"("path"=w611) -> ()
                          }
                          frame 1 {
                            n228 = Current VI's Path() -> (path=w613:path)
                            n229 = Strip Path(path=w613) -> (stripped path=w614:path)  [unwired: 1 out]
                            n230 = Build Path(base path=w614, name or relative path="1.wav" ("이름 또는 상대 경로")) -> (appended path=w612:path)
                            n231 = call "Sound_Sub.vi"("path"=w612) -> ()
                          }
                        }
                      }
                      frame Disabled {
                      }
                    }
                  }
                }
                n232 = global write "Control_Panel_정리.vi" "선택된 기능"(w528) -> ()
              }
              frame Enabled {
                n233 = case shown="참" w618 {
                  tunnel: w619 -> [_ w622]
                  tunnel: ["No Decesion" ("메시지") w621] -> w617
                  frame False {
                  }
                  frame True {
                    n234 = disable-structure shown="활성화" {
                      disable-tunnel: [w624 _ "" ("메시지")] -> w621
                      disable-tunnel: w622 -> [w623 w632 _]
                      frame Enabled {
                        n235 = case shown="5" w623 {
                          tunnel: ["온도" ("메시지") "자판" ("메시지") "침대" ("메시지") "용변" ("메시지") "기계" ("메시지") "응급" ("메시지") "No Decesion" ("메시지")] -> w624
                          frame 0 {
                          }
                          frame 1 {
                          }
                          frame 2 {
                          }
                          frame 3 {
                          }
                          frame 4 {
                          }
                          frame 5 {
                          }
                          frame 9, Default {
                          }
                        }
                      }
                      frame Disabled {
                        n236 = case shown="4" w632 {
                          frame 0, Default {
                            n237 = Current VI's Path() -> (path=w634:path)
                            n238 = Strip Path(path=w634) -> (stripped path=w635:path)  [unwired: 1 out]
                            n239 = Build Path(base path=w635, name or relative path="0.wav" ("이름 또는 상대 경로")) -> (appended path=w633:path)
                            n240 = call "Sound_Sub.vi"("path"=w633) -> ()
                          }
                          frame 2 {
                            n241 = Current VI's Path() -> (path=w637:path)
                            n242 = Strip Path(path=w637) -> (stripped path=w638:path)  [unwired: 1 out]
                            n243 = Build Path(base path=w638, name or relative path="2.wav" ("이름 또는 상대 경로")) -> (appended path=w640:path)
                            n244 = call "Sound_Sub.vi"("path"=w640) -> ()
                          }
                          frame 3 {
                            n245 = Current VI's Path() -> (path=w641:path)
                            n246 = Strip Path(path=w641) -> (stripped path=w642:path)  [unwired: 1 out]
                            n247 = Build Path(base path=w642, name or relative path="3.wav" ("이름 또는 상대 경로")) -> (appended path=w644:path)
                            n248 = call "Sound_Sub.vi"("path"=w644) -> ()
                          }
                          frame 4 {
                            n249 = Current VI's Path() -> (path=w645:path)
                            n250 = Strip Path(path=w645) -> (stripped path=w646:path)  [unwired: 1 out]
                            n251 = Build Path(base path=w646, name or relative path="4.wav" ("이름 또는 상대 경로")) -> (appended path=w648:path)
                            n252 = call "Sound_Sub.vi"("path"=w648) -> ()
                          }
                          frame 5 {
                            n253 = Current VI's Path() -> (path=w649:path)
                            n254 = Strip Path(path=w649) -> (stripped path=w650:path)  [unwired: 1 out]
                            n255 = Build Path(base path=w650, name or relative path="5.wav" ("이름 또는 상대 경로")) -> (appended path=w652:path)
                            n256 = call "Sound_Sub.vi"("path"=w652) -> ()
                          }
                          frame 1 {
                            n257 = Current VI's Path() -> (path=w654:path)
                            n258 = Strip Path(path=w654) -> (stripped path=w655:path)  [unwired: 1 out]
                            n259 = Build Path(base path=w655, name or relative path="1.wav" ("이름 또는 상대 경로")) -> (appended path=w653:path)
                            n260 = call "Sound_Sub.vi"("path"=w653) -> ()
                          }
                        }
                      }
                      frame Disabled {
                      }
                    }
                  }
                }
                n261 = global write "Control_Panel_정리.vi" "선택된 기능"(w617) -> ()
              }
            }
          }
        }
        n262 = global read "Control_Panel_정리.vi" "Random_num"() -> (w152:i32)
        n263 = global read "Control_Panel_정리.vi" "Experimentation_num"() -> (w153:i32)
        n264 = Multiply(x=w152, y=w153) -> (x*y=w151:i32)
        n265 = Subtract(x=w151, y=2) -> (x-y=w149:i32)
        n266 = Greater?(x=w132, y=w149) -> (0:w148:bool)
        n267 = Build Array (concatenate)(w100, w99) -> (w92:dbl[])
      }
    }
    frame #3 {
      n268 = disable-structure shown="Disabled" {
        disable-tunnel: w660 -> [w704 _]
        disable-tunnel: w659 -> [w703 _]
        frame Disabled {
          n269 = VISA Close(VISA resource name=w704, error in (no error)=w703) -> ()  [unwired: 1 out]
        }
        frame Enabled {
        }
      }
      n270 = dll-call lib="C:/Users/Server/Desktop/NeuroSky/NeuroSky_Dll_Call/Debug/NeuroSky_Dll_Call.dll" fn="FreeConnection"() -> ()  [unwired: 4 in, 2 out]
      n271 = global write "Control_Panel_정리.vi" "Acquisition Mode"(FALSE ("Device Control Enabled")) -> ()
      n272 = global write "Control_Panel_정리.vi" "Communication Stopped"(TRUE ("Device Control Enabled")) -> ()
      n273 = Build Path(base path=w663, name or relative path="Brain.txt") -> (appended path=w702:path)
      n274 = Build Path(base path=w663, name or relative path="selectedtarget.txt") -> (appended path=w694:path)
      n275 = Build Path(base path=w663, name or relative path="mius_flash_order.txt") -> (appended path=w699:path)
      n276 = Build Path(base path=w663, name or relative path="Target_order.txt") -> (appended path=w689:path)
      n277 = Build Path(base path=w663, name or relative path="Accuracy.txt") -> (appended path=w692:path)
      n278 = Build Path(base path=w663, name or relative path="ERP_발생_total.txt") -> (appended path=w682:path)
      n279 = Build Path(base path=w663, name or relative path="ERP_all_icon.txt") -> (appended path=w678:path)
      n280 = Build Path(base path=w663, name or relative path="ERP_total.txt") -> (appended path=w666:path)
      n281 = Build Path(base path=w663, name or relative path="SWLDA_hyperplane_value.txt") -> (appended path=w674:path)
      n282 = Build Path(base path=w663, name or relative path="decision_value.txt") -> (appended path=w671:path)
      n283 = call-poly <vilib>:"Write To Spreadsheet File.vi"("format (%.3f)"="%.6f", "1D data"=w658, "file path (dialog if empty)"=w702) -> ()  [unwired: 5 in, 1 out]
      n284 = call-poly <vilib>:"Write To Spreadsheet File.vi"("1D data"=w693, "file path (dialog if empty)"=w694) -> ()  [unwired: 6 in, 1 out]
      n285 = call-poly <vilib>:"Write To Spreadsheet File.vi"("transpose? (no:F)"=TRUE, "2D data"=w697, "file path (dialog if empty)"=w699) -> ()  [unwired: 5 in, 1 out]
      n286 = call-poly <vilib>:"Write To Spreadsheet File.vi"("transpose? (no:F)"=TRUE, "1D data"=w686, "file path (dialog if empty)"=w689) -> ()  [unwired: 5 in, 1 out]
      n287 = call-poly <vilib>:"Write To Spreadsheet File.vi"("1D data"=w690, "file path (dialog if empty)"=w692) -> ()  [unwired: 6 in, 1 out]
      n288 = call-poly <vilib>:"Write To Spreadsheet File.vi"("transpose? (no:F)"=TRUE, "1D data"=w680, "file path (dialog if empty)"=w682) -> ()  [unwired: 5 in, 1 out]
      n289 = call-poly <vilib>:"Write To Spreadsheet File.vi"("transpose? (no:F)"=TRUE, "format (%.3f)"="%.6f", "2D data"=w675, "file path (dialog if empty)"=w678) -> ()  [unwired: 4 in, 1 out]
      n290 = call-poly <vilib>:"Write To Spreadsheet File.vi"("transpose? (no:F)"=TRUE, "format (%.3f)"="%.6f", "2D data"=w664, "file path (dialog if empty)"=w666) -> ()  [unwired: 4 in, 1 out]
      n291 = call-poly <vilib>:"Write To Spreadsheet File.vi"("format (%.3f)"="%.6f", "1D data"=w672, "file path (dialog if empty)"=w674) -> ()  [unwired: 5 in, 1 out]
      n292 = call-poly <vilib>:"Write To Spreadsheet File.vi"("format (%.3f)"="%.6f", "1D data"=w669, "file path (dialog if empty)"=w671) -> ()  [unwired: 5 in, 1 out]
    }
    frame #4 {
      n293 = global write "Control_Panel_정리.vi" "Communication Stopped"(FALSE ("Device Control Enabled")) -> ()
    }
  }
